vi "Is Caraya Unit Test.vi"(8 "Error in":errorcluster caption="Error in (no error)", 10 "VI Path":path, 11 "DMC Test Runner in":refnum<class "DMC Test Runner.lvclass">) -> (0 "Error out":errorcluster, 2 "Contains Define Test.vi?":bool, 3 "DMC Test Runner out":refnum<class "DMC Test Runner.lvclass">)   [LabVIEW 2023, in "DMC Test Runner.lvclass"]
uses:
  DMC Test Runner.lvclass
  C:/Program Files/National Instruments/LabVIEW 2023/vi.lib/addons/_JKI Toolkits/Caraya/classes/Test Runner/Test Runner.lvclass
  DMC Test Runner.lvclass/DMC Test Runner.ctl
  <vilib>/Utility/traverseref.llb/TRef TravTarget.ctl
  <vilib>/addons/_JKI Toolkits/Caraya/classes/Test/Define Test.vi
  <vilib>/addons/_JKI Toolkits/Caraya/classes/Test/Test.lvclass
  <vilib>/addons/_JKI Toolkits/Caraya/classes/Test Runner/Test Runner.lvclass
  <vilib>/Utility/traverseref.llb/VI Scripting - Traverse.lvlib
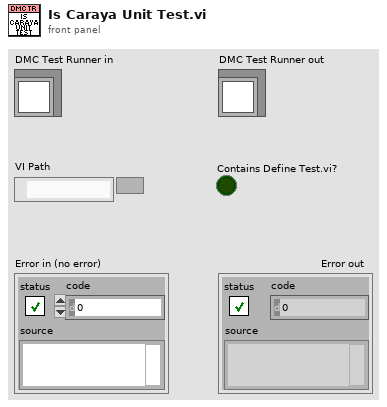
[diagram p1: front panel]
types:
  T1 = typedef "TRef TravTarget.ctl" = enum16{"FP", "BD", "Other"}
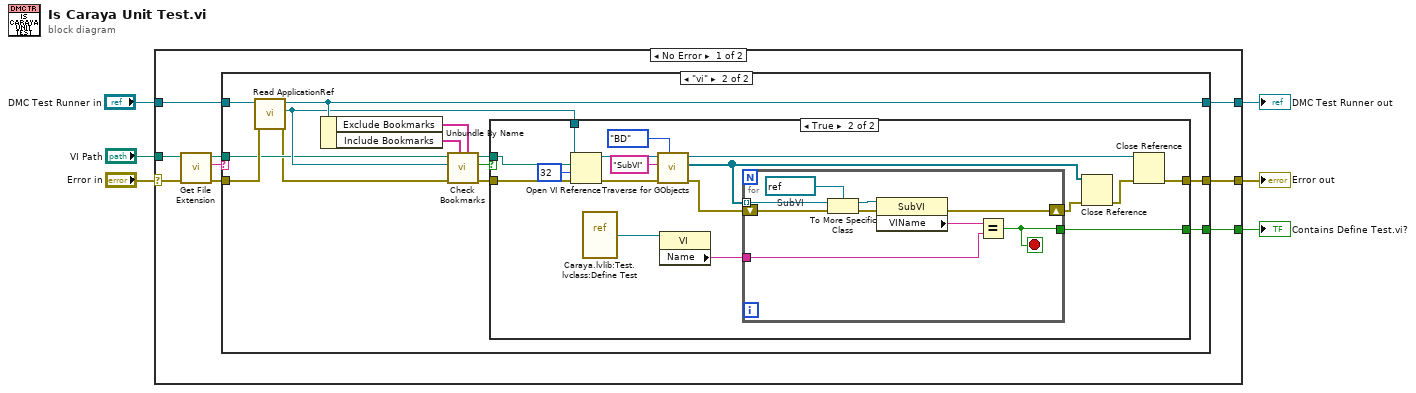
[diagram p0: block diagram]
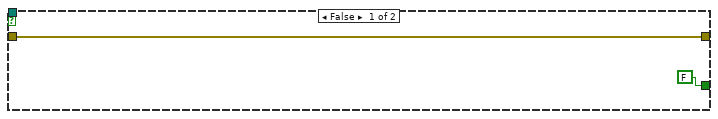
[diagram p3: hidden frame]
diagram:
  n1 = case shown="No Error" "Error in" {
    selector: "Error in" -> [w12 w60]
    tunnel: [w15 w60] -> w6
    tunnel: [w14 _] -> w5
    tunnel: "VI Path" -> [w13 _]
    tunnel: "DMC Test Runner in" -> [w8 w59]
    tunnel: [w7 w59] -> w1
    frame No Error {
      n2 = call <vilib>:"Get File Extension.vi"("error in (no error)"=w12, "file"=w13) -> ("error out"=w11:errorcluster, "lowercase file extension"=w9:string, "dup file"=w10:path)  [unwired: 5 in, 2 out]
      n3 = case shown="\"vi\"" w9 {
        tunnel: [w17 w30] -> w15
        tunnel: [_ w29] -> w14
        tunnel: w11 -> [w17 w28]
        tunnel: w10 -> [_ w22]
        tunnel: w8 -> [w16 w27]
        tunnel: [w16 w26] -> w7
        frame Default {
        }
        frame "vi" {
          n4 = call <vilib>:"Read ApplicationRef.vi"("error in (no error)"=w28, "Test Runner in"=w27) -> ("error out"=w19:errorcluster, "Application"=w23:refnum<vi>, "Test Runner out"=w26:refnum<class "DMC Test Runner.lvclass">)  [unwired: 7 in]
          n5 = Unbundle By Name(w26) -> ("Exclude Bookmarks"=w24:string[], "Include Bookmarks"=w25:string[])
          n6 = call "Check Bookmarks.vi"("Exclude Bookmarks"=w24, "Include Bookmarks"=w25, "error in (no error)"=w19, "App Ref"=w23, "VI Path"=w22) -> ("error out"=w18:errorcluster, "Check If Unit Test?"=w20:bool, "VI Path dup"=w21:path)  [unwired: 4 in]
          n7 = case shown="True" w20 {
            tunnel: [w32 w49] -> w30
            tunnel: [FALSE w48] -> w29
            tunnel: w18 -> [w32 w47]
            tunnel: w23 -> [_ w43]
            tunnel: w21 -> [_ w42]
            frame False {
            }
            frame True {
              n8 = Open VI Reference(application reference (local)=w43, vi path=w42, options=32, error in (no error)=w47) -> (vi reference=w40:refnum<vi>, error out=w41:errorcluster)  [unwired: 2 in]
              n9 = vi-ref "Caraya.lvlib:Test.lvclass:Define Test.vi"() -> (w46:refnum<vi>)
              n10 = call <vilib>:"Traverse for GObjects.vi"("Traverse Target"=TRef_TravTarget."BD", "error in (no error)"=w41, "Class Name"="SubVI", "VI Refnum"=w40) -> ("error out"=w36:errorcluster, "References"=w35:refnum<vi>[], "dup VI Refnum"=w37:refnum<vi>)  [unwired: 4 in, 1 out]
              n11 = property class="VI"(reference=w46) -> ("Name"=w45:string)  [unwired: 1 in, 2 out]
              n12 = for {
                tunnel: w35 -> [w58] mode=indexing
                tunnel: w45 -> [w55]
                shift-right: [w56] -> w44
                shift-left: w36 -> [w57]
                tunnel: [w54] -> w48
                stop <- w54 stop-if-true
                w53 = refnum<vi> refnum  # SubVI
                n13 = To More Specific Class(target class=w53, reference=w58, error in=w57) -> (specific class reference=w52:refnum<vi>, error out=w51:errorcluster)
                n14 = property class="SubVI"(reference=w52, error in=w51) -> (error out=w56:errorcluster, "VIName"=w50:string)  [unwired: 1 out]
                n15 = Equal?(x=w50, y=w55) -> (x = y?=w54:bool)
              }
              n16 = Close Reference(reference=w35, error in (no error)=w44) -> (error out=w34:errorcluster)
              n17 = Close Reference(reference=w37, error in (no error)=w34) -> (error out=w49:errorcluster)
            }
          }
        }
      }
    }
    frame Error {
    }
  }
  "Error out" <- w6
  "Contains Define Test.vi?" <- w5
  "DMC Test Runner out" <- w1
